vi "Drive set.vi"(0 "Drive Global Data":T1) -> ()   [LabVIEW 2013]
uses:
  <vilib>/Rock Robotics/WPI/RobotDrive/WPI_RobotDriveArcadeDrive_Standard(NoSaturation).vi
  <vilib>/Rock Robotics/WPI/RobotDrive/WPI_RobotDriveGetSetRefNum.vi
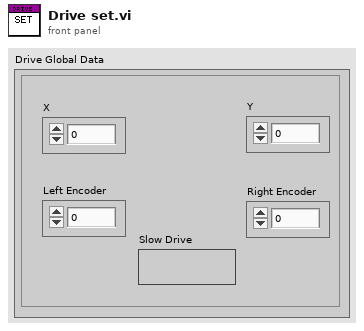
[diagram p1: front panel]
types:
  T1 = cluster{"Y":dbl, "X":dbl, "Left Encoder":dbl, "Right Encoder":dbl, "Slow Drive":bool}
  T2 = typedef "WPI_RobotDriveDevRef.ctl" = cluster{"DevStatus":errorcluster, "Motors[]":T3[], "Square Inputs":bool, "Max Output":dbl, "Isochronous":bool}
  T3 = typedef "WPI_MotorControlDeviceRef.ctl" = cluster{"DeviceStatus":errorcluster, "Type":enum16{"PWM", "CAN"}, "PWM":cluster{"Digital Module":T4, "PWM Channel":T5, "DeadBand":T6}, "CAN":cluster{"Device Number":u8, "Control Mode":T7, "Semaphore":T8, "Max Vout":dbl}, "Invert":bool, "TransformRef":T9, "InvTransformRef":T9}
  T4 = typedef "FPGA_TypedefDigitalModule.ctl" = enum16{"Digital Module 1", "Digital Module 2"}
  T5 = typedef "FPGA_DIOPWMChannel.ctl" = enum8{"PWM 1", "PWM 2", "PWM 3", "PWM 4", "PWM 5", "PWM 6", "PWM 7", "PWM 8", "PWM 9", "PWM 10", "Invalid"}
  T6 = typedef "WPI_PWMDeadband.ctl" = cluster{"Name":string, "maxPositivePwm":i32, "minPositivePwm":i32, "centerPwm":i32, "maxNegativePwm":i32, "minNegativePwm":i32, "angularRange":u16}
  T7 = typedef "WPI_CANJaguar_ControlMode.ctl" = enum8{"Percent VBus", "Current", "Speed", "Position", "Voltage"}
  T8 = typedef "Semaphore RefNum" = refnum<k1>
  T9 = typedef "WPI_PWMTransform_ConPane.ctl" = refnum<vi>
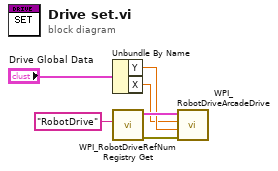
[diagram p0: block diagram]
diagram:
  n1 = Unbundle By Name("Drive Global Data") -> ("Y"=w2:dbl, "X"=w1:dbl)
  n2 = call <vilib>:"WPI_RobotDriveRefNum Registry Get.vi"("refnum name"="RobotDrive") -> ("error out"=w4:errorcluster, "RobotDriveDevRef"=w5:T2)  [unwired: 9 in]
  n3 = call-poly <vilib>:"WPI_RobotDriveArcadeDrive.vi"("error in (no error)"=w4, "Y axis value"=w2, "X axis value"=w1, "RobotDriveDevRef"=w5) -> ()  [unwired: 5 in, 3 out]
